vi "QuadratureEncoder.vi"(3 "Reset":bool, 4 "TimerConfig":T2, 5 "AnalogTriggers":T1[](array[typedef])=[{"InHysteresis"=FALSE, "OverLimit"=FALSE, "Rising"=FALSE, "Falling"=FALSE}, {"InHysteresis"=FALSE, "OverLimit"=FALSE, "Rising"=FALSE, "Falling"=FALSE}, {"InHysteresis"=FALSE, "OverLimit"=FALSE, "Rising"=FALSE, "Falling"=FALSE}, {"InHysteresis"=FALSE, "OverLimit"=FALSE, "Rising"=FALSE, "Falling"=FALSE}, {"InHysteresis"=FALSE, "OverLimit"=FALSE, "Rising"=FALSE, "Falling"=FALSE}, {"InHysteresis"=FALSE, "OverLimit"=FALSE, "Rising"=FALSE, "Falling"=FALSE}, {"InHysteresis"=FALSE, "OverLimit"=FALSE, "Rising"=FALSE, "Falling"=FALSE}, {"InHysteresis"=FALSE, "OverLimit"=FALSE, "Rising"=FALSE, "Falling"=FALSE}], 6 "DigitalInputs":bool[](array[boolean])=[FALSE, FALSE, FALSE, FALSE, FALSE, FALSE, FALSE, FALSE, FALSE, FALSE, FALSE, FALSE, FALSE, FALSE, FALSE, FALSE, FALSE, FALSE, FALSE, FALSE, FALSE, FALSE, FALSE, FALSE, FALSE, FALSE, FALSE, FALSE, FALSE, FALSE, FALSE, FALSE], 7 "Config":T4) -> (0 "TimerOutput":cluster{"Period":u32, "Stopped":bool}, 1 "Output":T5)   [LabVIEW 2019]
uses:
  Helpers/Source.ctl
  Helpers/AnalogTriggerOutput.ctl
  <vilib>/rvi/Emulation/niFpgaSctlEmulationGetInTimedLoop.vi
  <vilib>/rvi/Emulation/niFpgaProcessEmulError.vi
  <vilib>/rvi/FXPMathLib/FxpAdd/XNode/nifxpmath_Add.xnode
  <vilib>/rvi/FXPMathLib/sim/FxpSim.dll
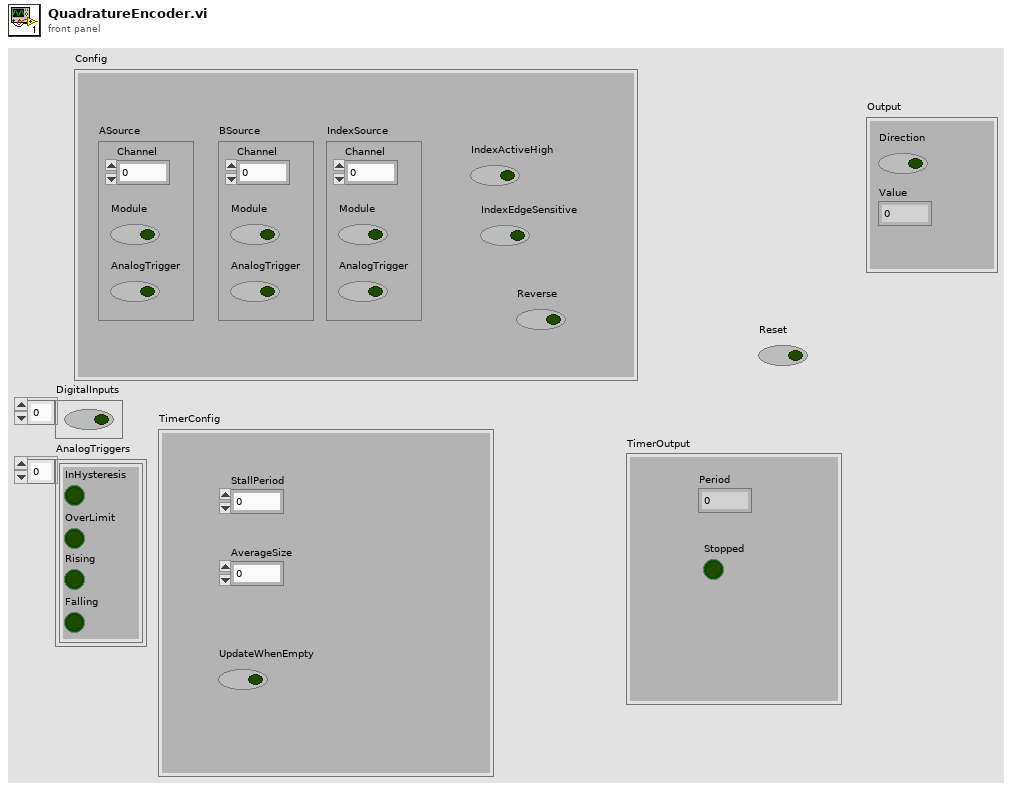
[diagram p1: front panel]
types:
  T1 = typedef "AnalogTriggerOutput.ctl" = cluster{"InHysteresis":bool, "OverLimit":bool, "Rising":bool, "Falling":bool}
  T2 = cluster{"StallPeriod":fxp<+,24,24>, "AverageSize":fxp<+,7,7>, "UpdateWhenEmpty":bool}
  T3 = typedef "Source.ctl" = cluster{"Channel":fxp<+,4,4>, "Module":bool, "AnalogTrigger":bool}
  T4 = cluster{"ASource":T3, "BSource":T3, "IndexSource":T3, "IndexActiveHigh":bool, "IndexEdgeSensitive":bool, "Reverse":bool}
  T5 = cluster{"Direction":bool, "Value":fxp<+/-,31,31>}
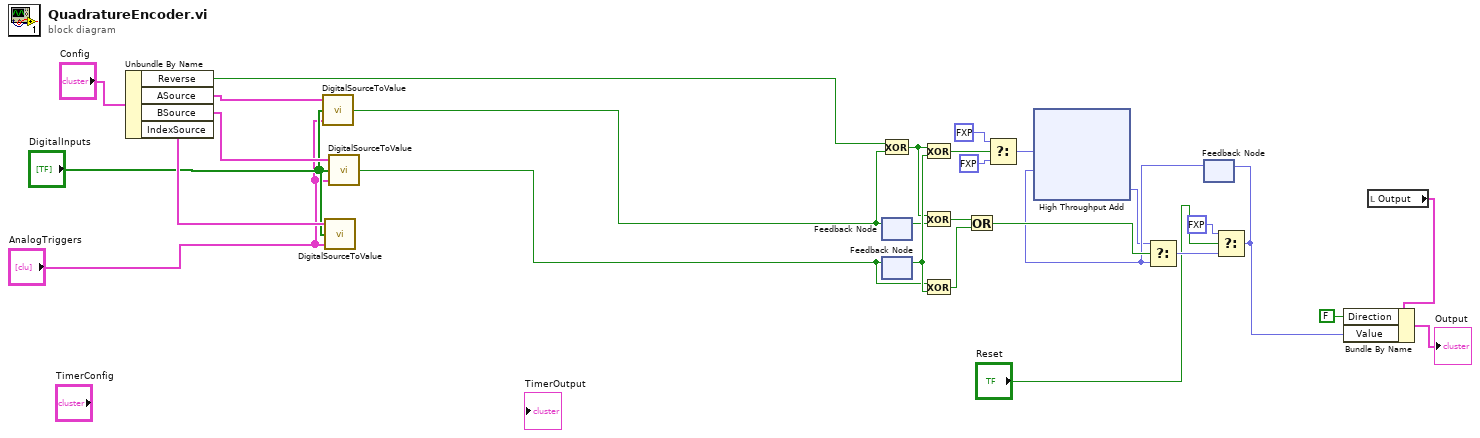
[diagram p0: block diagram]
diagram:
  n1 = Unbundle By Name("Config") -> ("Reverse"=w7:bool, "ASource"=w13:T3, "BSource"=w12:T3, "IndexSource"=w11:T3)
  n2 = call "DigitalSourceToValue.vi"("AnalogTriggers"="AnalogTriggers", "DigitalInputs"="DigitalInputs", "Source"=w13) -> ("Value"=w9:bool)
  n3 = call "DigitalSourceToValue.vi"("AnalogTriggers"="AnalogTriggers", "DigitalInputs"="DigitalInputs", "Source"=w11) -> ()  [unwired: 1 out]
  n4 = call "DigitalSourceToValue.vi"("AnalogTriggers"="AnalogTriggers", "DigitalInputs"="DigitalInputs", "Source"=w12) -> ("Value"=w8:bool)
  n5 = Exclusive Or(1:w9, 2:w7) -> (0:w22:bool)
  n6 = feedback-in #1(w9) -> ()
  n7 = feedback #1() -> (w23:bool)  [unwired: 1 in]
  n8 = feedback #2() -> (w24:bool)  [unwired: 1 in]
  n9 = feedback-in #2(w8) -> ()
  n10 = Exclusive Or(1:w24, 2:w22) -> (0:w28:bool)
  n11 = Exclusive Or(1:w23, 2:w22) -> (0:w27:bool)
  n12 = Exclusive Or(1:w24, 2:w8) -> (0:w26:bool)
  n13 = Or(x=w27, y=w26) -> (x .or. y?=w25:bool)
  n14 = Select(t=fxp<+/-,31,31> 1.0 ("Count"), s=w28, f=fxp<+/-,31,31> -1.0 ("Count")) -> (s? t:f=w17:fxp<+/-,31,31>)
  n15 = feedback #3() -> (w16:fxp<+/-,31,31>)  [unwired: 1 in]
  n16 = xnode ("High Throughput Add")("x"=w17, "y"=w16) -> ("x+y"=w15:fxp<+/-,31,31>)
  n17 = Select(t=w15, s=w25, f=w16) -> (s? t:f=w18:fxp<+/-,31,31>)
  n18 = Select(t=fxp<+/-,31,31> 0.0 ("Count"), s="Reset", f=w18) -> (s? t:f=w2:fxp<+/-,31,31>)
  n19 = feedback-in #3(w2) -> ()
  n20 = local read "Output"() -> (w5:T5)
  n21 = Bundle By Name(cluster=w5, "Direction"=FALSE, "Value"=w2) -> (→"Output":T5)
